vi "StartUp Sequence Open Loop Rev 1.1.vi"() -> ()   [LabVIEW 2017]
panel:
  in  "Shut Off":bool
  out "ECU COM Port Out":refnum<visa-resource-name>
  out "Throttle Position":string
  out "Turbine RPM":string
  out "Turbine Temp":string
  out "Pump Voltage":string
  out "Error Out":errorcluster
  in  "Error In":errorcluster
  in  "ECU COM Port":refnum<visa-resource-name>
  out "Turbine State":string
  in  "Strt Sqnc":bool
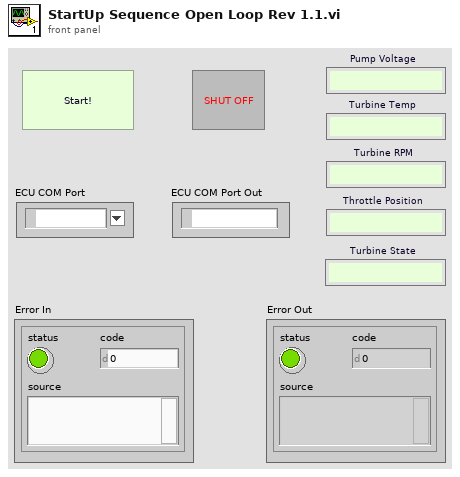
[diagram p1: front panel]
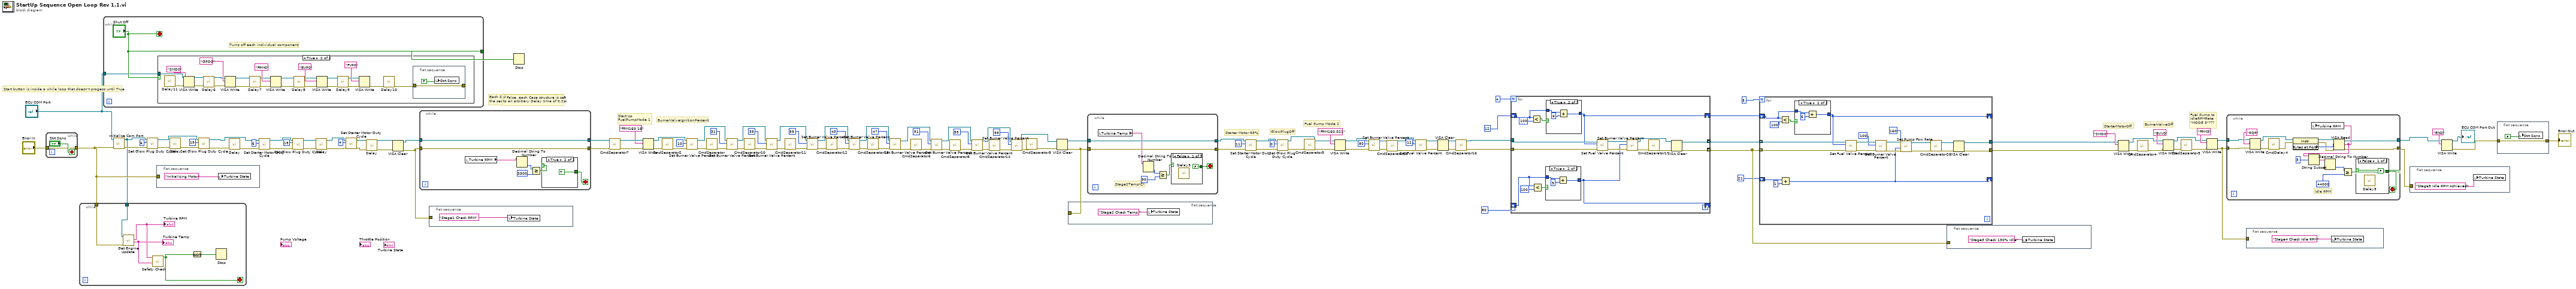
[diagram p0: block diagram]
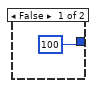
[diagram p2: hidden frame]
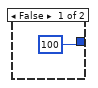
[diagram p3: hidden frame]
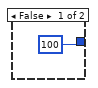
[diagram p4: hidden frame]
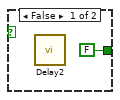
[diagram p6: hidden frame]
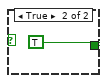
[diagram p7: hidden frame]
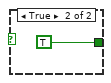
[diagram p8: hidden frame]
diagram:
  # "Start button is inside a while loop that doesn't progess until True"
  # "Fuel Pump Mode 2"
  # "Starter Motor 55%"
  # "Fuel Pump to \nIdleRPMRate\n\"MODE 3\"???"
  # "BurnerValveOff"
  # "StarterMotorOff"
  # "GlowPlugOff"
  # "Start Up\nFuelPumpMode 1"
  # "BurnerValveIgnitionPercent"
  # "If False, each Case structure is set\nto an arbitrary Delay time of 0.2 s"
  # "Each Stage is inside a while loop so that \nthe sequence doesn't progress until True"
  n1 = while {
    tunnel: "Error In" -> [w122]
    tunnel: [w122] -> w2
    stop <- "Strt Sqnc" stop-if-true
  }
  n2 = while {
    tunnel: ["Shut Off"] -> w94
    tunnel: "ECU COM Port" -> [w124]
    stop <- "Shut Off" stop-if-true
    # "Turns off each individual component"
    n3 = case shown="True" "Shut Off" {
      tunnel: w124 -> [_ w128]
      frame False {
      }
      frame True {
        n4 = call "Delay11"() -> ("error out"=w126:errorcluster)  [unwired: 11 in]
        n5 = VISA Write(VISA resource name=w128, write buffer="SMD0", error in (no error)=w126) -> (VISA resource name out=w133:refnum<visa-resource-name>, error out=w146:errorcluster)  [unwired: 1 out]
        n6 = call "Delay6"("error in (no error)"=w146) -> ("error out"=w140:errorcluster)  [unwired: 10 in]
        n7 = VISA Write(VISA resource name=w133, write buffer="GPD0", error in (no error)=w140) -> (VISA resource name out=w131:refnum<visa-resource-name>, error out=w144:errorcluster)  [unwired: 1 out]
        n8 = call "Delay7"("error in (no error)"=w144) -> ("error out"=w139:errorcluster)  [unwired: 10 in]
        n9 = VISA Write(VISA resource name=w131, write buffer="FPM0", error in (no error)=w139) -> (VISA resource name out=w130:refnum<visa-resource-name>, error out=w143:errorcluster)  [unwired: 1 out]
        n10 = call "Delay8"("error in (no error)"=w143) -> ("error out"=w138:errorcluster)  [unwired: 10 in]
        n11 = VISA Write(VISA resource name=w130, write buffer="BVP0", error in (no error)=w138) -> (VISA resource name out=w129:refnum<visa-resource-name>, error out=w142:errorcluster)  [unwired: 1 out]
        n12 = call "Delay9"("error in (no error)"=w142) -> ("error out"=w137:errorcluster)  [unwired: 10 in]
        n13 = VISA Write(VISA resource name=w129, write buffer="FVP0", error in (no error)=w137) -> (error out=w141:errorcluster)  [unwired: 2 out]
        n14 = call "Delay10"("error in (no error)"=w141) -> ("error out"=w127:errorcluster)  [unwired: 10 in]
        n15 = flat-sequence {
          tunnel: w127 -> [w147]
          tunnel: [w147] -> _
          frame #0 {
            n16 = local write "Strt Sqnc"(FALSE ("Strt Sqnc")) -> ()
          }
        }
      }
    }
  }
  n17 = call "Initialize Com Port.vi"("Error In"=w2, "ECU COM Port"="ECU COM Port") -> ("Error Out"=w82:errorcluster, "ECU COM Port Out"=w1:refnum<visa-resource-name>)  [unwired: 8 in]
  n18 = while {
    tunnel: w2 -> [w154]
    tunnel: w1 -> [w153]
    stop <- w150 stop-if-true
    n19 = call "Get Engine Update.vi"("Error In"=w154, "ECU COM Port"=w153) -> ("Temperature"=w151:string, "RPMs"=w152:string)  [unwired: 6 in, 2 out]
    "Turbine RPM" <- w152
    "Turbine Temp" <- w151
    n20 = call "Safety Check.vi"("Temperature"=w151, "RPMs"=w152) -> ("Safe?"=w150:bool)  [unwired: 9 in]
    n21 = Not(x=w150) -> (.not. x?=w149:bool)
    n22 = Stop(stop? (T)=w149) -> ()
  }
  n23 = call "Set Glow Plug Duty Cycle.vi"("Error In"=w82, "Duty Cycle"=6, "ECU COM Port"=w1) -> ("Error Out"=w81:errorcluster, "ECU COM Port Out"=w78:refnum<visa-resource-name>)  [unwired: 7 in]
  n24 = flat-sequence {
    tunnel: w2 -> [_]
    frame #0 {
      n25 = local write "Turbine State"("Initializing Motor") -> ()
    }
  }
  n26 = call "Delay"("error in (no error)"=w81) -> ("error out"=w80:errorcluster)  [unwired: 10 in]
  n27 = call "Set Glow Plug Duty Cycle.vi"("Error In"=w80, "Duty Cycle"=19, "ECU COM Port"=w78) -> ("Error Out"=w79:errorcluster, "ECU COM Port Out"=w74:refnum<visa-resource-name>)  [unwired: 7 in]
  n28 = call "Delay"("error in (no error)"=w79) -> ("error out"=w75:errorcluster)  [unwired: 10 in]
  n29 = call "Set Starter Motor Duty Cycle.vi"("Error In"=w75, "Duty Cycle"=6, "ECU COM Port"=w74) -> ("Error Out"=w73:errorcluster, "ECU COM Port Out"=w71:refnum<visa-resource-name>)  [unwired: 7 in]
  n30 = call "Set Glow Plug Duty Cycle.vi"("Error In"=w73, "Duty Cycle"=15, "ECU COM Port"=w71) -> ("Error Out"=w72:errorcluster, "ECU COM Port Out"=w67:refnum<visa-resource-name>)  [unwired: 7 in]
  n31 = call "Delay"("error in (no error)"=w72) -> ("error out"=w69:errorcluster)  [unwired: 10 in]
  n32 = call "Set Starter Motor Duty Cycle.vi"("Error In"=w69, "Duty Cycle"=4, "ECU COM Port"=w67) -> ("Error Out"=w68:errorcluster, "ECU COM Port Out"=w66:refnum<visa-resource-name>)  [unwired: 7 in]
  n33 = call "Delay"("error in (no error)"=w68) -> ("error out"=w97:errorcluster)  [unwired: 10 in]
  n34 = VISA Clear(VISA resource name=w66, error in (no error)=w97) -> (VISA resource name out=w98:refnum<visa-resource-name>, error out=w99:errorcluster)
  n35 = while {
    tunnel: w99 -> [w158]
    tunnel: w98 -> [w157]
    tunnel: [w157] -> w109
    tunnel: [w158] -> w108
    stop <- w161 stop-if-true
    n36 = local read "Turbine RPM"() -> (w156:string)
    n37 = Decimal String To Number(string=w156) -> (number=w160:i32)  [unwired: 2 in, 1 out]
    n38 = Greater Or Equal?(x=w160, y=3300) -> (x >= y?=w162:bool)
    n39 = case shown="True" w162 {
      tunnel: [FALSE TRUE] -> w161
      frame False {
        n40 = call "Delay2"() -> ()  [unwired: 11 in, 1 out]
      }
      frame True {
      }
    }
  }
  n41 = flat-sequence {
    tunnel: w99 -> [_]
    frame #0 {
      n42 = local write "Turbine State"("Stage1 Check RPM") -> ()
    }
  }
  n43 = Stop(stop? (T)=w94) -> ()
  n44 = call "CmdSeparator7"("error in (no error)"=w108) -> ("error out"=w107:errorcluster)  [unwired: 10 in]
  n45 = VISA Write(VISA resource name=w109, write buffer="FPM160,16", error in (no error)=w107) -> (VISA resource name out=w54:refnum<visa-resource-name>, error out=w120:errorcluster)  [unwired: 1 out]
  n46 = call "CmdSeparator2"("error in (no error)"=w120) -> ("error out"=w65:errorcluster)  [unwired: 10 in]
  n47 = call "Set Burner Valve Percent.vi"("Error In"=w65, "Percent"=10, "ECU COM Port"=w54) -> ("Error Out"=w64:errorcluster, "ECU COM Port Out"=w53:refnum<visa-resource-name>)  [unwired: 7 in]
  n48 = call "CmdSeparator"("error in (no error)"=w64) -> ("error out"=w63:errorcluster)  [unwired: 10 in]
  n49 = call "Set Burner Valve Percent.vi"("Error In"=w63, "Percent"=31, "ECU COM Port"=w53) -> ("Error Out"=w62:errorcluster, "ECU COM Port Out"=w52:refnum<visa-resource-name>)  [unwired: 7 in]
  n50 = call "CmdSeparator10"("error in (no error)"=w62) -> ("error out"=w61:errorcluster)  [unwired: 10 in]
  n51 = call "Set Burner Valve Percent.vi"("Error In"=w61, "Percent"=35, "ECU COM Port"=w52) -> ("Error Out"=w60:errorcluster, "ECU COM Port Out"=w51:refnum<visa-resource-name>)  [unwired: 7 in]
  n52 = call "CmdSeparator11"("error in (no error)"=w60) -> ("error out"=w59:errorcluster)  [unwired: 10 in]
  n53 = call "Set Burner Valve Percent.vi"("Error In"=w59, "Percent"=39, "ECU COM Port"=w51) -> ("Error Out"=w58:errorcluster, "ECU COM Port Out"=w50:refnum<visa-resource-name>)  [unwired: 7 in]
  n54 = call "CmdSeparator12"("error in (no error)"=w58) -> ("error out"=w57:errorcluster)  [unwired: 10 in]
  n55 = call "Set Burner Valve Percent.vi"("Error In"=w57, "Percent"=43, "ECU COM Port"=w50) -> ("Error Out"=w56:errorcluster, "ECU COM Port Out"=w49:refnum<visa-resource-name>)  [unwired: 7 in]
  n56 = call "CmdSeparator13"("error in (no error)"=w56) -> ("error out"=w55:errorcluster)  [unwired: 10 in]
  n57 = call "Set Burner Valve Percent.vi"("Error In"=w55, "Percent"=47, "ECU COM Port"=w49) -> ("Error Out"=w25:errorcluster, "ECU COM Port Out"=w24:refnum<visa-resource-name>)  [unwired: 7 in]
  n58 = call "CmdSeparator6"("error in (no error)"=w25) -> ("error out"=w27:errorcluster)  [unwired: 10 in]
  n59 = call "Set Burner Valve Percent.vi"("Error In"=w27, "Percent"=51, "ECU COM Port"=w24) -> ("Error Out"=w20:errorcluster, "ECU COM Port Out"=w21:refnum<visa-resource-name>)  [unwired: 7 in]
  n60 = call "CmdSeparator8"("error in (no error)"=w20) -> ("error out"=w23:errorcluster)  [unwired: 10 in]
  n61 = call "Set Burner Valve Percent.vi"("Error In"=w23, "Percent"=55, "ECU COM Port"=w21) -> ("Error Out"=w16:errorcluster, "ECU COM Port Out"=w17:refnum<visa-resource-name>)  [unwired: 7 in]
  n62 = call "CmdSeparator14"("error in (no error)"=w16) -> ("error out"=w19:errorcluster)  [unwired: 10 in]
  n63 = call "Set Burner Valve Percent.vi"("Error In"=w19, "Percent"=59, "ECU COM Port"=w17) -> ("Error Out"=w15:errorcluster, "ECU COM Port Out"=w14:refnum<visa-resource-name>)  [unwired: 7 in]
  n64 = call "CmdSeparator9"("error in (no error)"=w15) -> ("error out"=w93:errorcluster)  [unwired: 10 in]
  n65 = VISA Clear(VISA resource name=w14, error in (no error)=w93) -> (VISA resource name out=w95:refnum<visa-resource-name>, error out=w96:errorcluster)
  n66 = flat-sequence {
    tunnel: w96 -> [_]
    frame #0 {
      n67 = local write "Turbine State"("Stage2 Check Temp.") -> ()
    }
  }
  n68 = while {
    tunnel: w95 -> [w168]
    tunnel: w96 -> [w169]
    tunnel: [w168] -> w36
    tunnel: [w169] -> w38
    stop <- w172 stop-if-true
    # "Stage2Temp(C)"
    n69 = local read "Turbine Temp"() -> (w167:string)
    n70 = Decimal String To Number(string=w167) -> (number=w170:i32)  [unwired: 2 in, 1 out]
    n71 = Greater Or Equal?(x=w170, y=90) -> (x >= y?=w173:bool)
    n72 = case shown="False" w173 {
      tunnel: [FALSE TRUE] -> w172
      frame False {
        n73 = call "Delay3"() -> ()  [unwired: 11 in, 1 out]
      }
      frame True {
      }
    }
  }
  n74 = call "Set Starter Motor Duty Cycle.vi"("Error In"=w38, "Duty Cycle"=11, "ECU COM Port"=w36) -> ("Error Out"=w37:errorcluster, "ECU COM Port Out"=w35:refnum<visa-resource-name>)  [unwired: 7 in]
  n75 = call "Set Glow Plug Duty Cycle.vi"("Error In"=w37, "Duty Cycle"=0, "ECU COM Port"=w35) -> ("Error Out"=w34:errorcluster, "ECU COM Port Out"=w32:refnum<visa-resource-name>)  [unwired: 7 in]
  n76 = call "CmdSeparator3"("error in (no error)"=w34) -> ("error out"=w33:errorcluster)  [unwired: 10 in]
  n77 = VISA Write(VISA resource name=w32, write buffer="FPM160,021", error in (no error)=w33) -> (VISA resource name out=w29:refnum<visa-resource-name>, error out=w31:errorcluster)  [unwired: 1 out]
  n78 = call "Set Burner Valve Percent.vi"("Error In"=w31, "Percent"=80, "ECU COM Port"=w29) -> ("Error Out"=w13:errorcluster, "ECU COM Port Out"=w28:refnum<visa-resource-name>)  [unwired: 7 in]
  n79 = call "CmdSeparator18"("error in (no error)"=w13) -> ("error out"=w12:errorcluster)  [unwired: 10 in]
  n80 = call "Set Fuel Valve Percent.vi"("Error In"=w12, "Percent"=12, "ECU COM Port"=w28) -> ("Error Out"=w11:errorcluster, "ECU COM Port Out"=w30:refnum<visa-resource-name>)  [unwired: 7 in]
  n81 = VISA Clear(VISA resource name=w30, error in (no error)=w11) -> (VISA resource name out=w89:refnum<visa-resource-name>, error out=w90:errorcluster)
  n82 = call "CmdSeparator16"("error in (no error)"=w90) -> ("error out"=w88:errorcluster)  [unwired: 10 in]
  n83 = for {
    N: 4 -> [_]
    tunnel: [w176] -> _
    tunnel: [w177] -> _
    tunnel: w89 -> [w184]
    tunnel: w88 -> [w185]
    shift-right: [w183] -> w6
    shift-left: 12 -> [w189]
    shift-right: [w180] -> _
    shift-left: 80 -> [w186]
    tunnel: [w177] -> w8 mode=indexing
    tunnel: [w176] -> w7 mode=indexing
    n84 = Less?(x=w189, y=100) -> (x < y?=w190:bool)
    n85 = Less?(x=w186, y=100) -> (x < y?=w187:bool)
    n86 = case shown="True" w187 {
      tunnel: w186 -> [_ w196]
      tunnel: [100 w194] -> w180
      frame False {
      }
      frame True {
        n87 = Add(x=w196, y=5) -> (x+y=w194:i32)
      }
    }
    n88 = case shown="True" w190 {
      tunnel: w189 -> [_ w200]
      tunnel: [100 w198] -> w183
      frame False {
      }
      frame True {
        n89 = Add(x=w200, y=6) -> (x+y=w198:i32)
      }
    }
    n90 = call "Set Fuel Valve Percent.vi"("Error In"=w185, "Percent"=w183, "ECU COM Port"=w184) -> ("Error Out"=w182:errorcluster, "ECU COM Port Out"=w179:refnum<visa-resource-name>)  [unwired: 7 in]
    n91 = call "Set Burner Valve Percent.vi"("Error In"=w182, "Percent"=w180, "ECU COM Port"=w179) -> ("Error Out"=w181:errorcluster, "ECU COM Port Out"=w178:refnum<visa-resource-name>)  [unwired: 7 in]
    n92 = call "CmdSeparator17"("error in (no error)"=w181) -> ("error out"=w192:errorcluster)  [unwired: 10 in]
    n93 = VISA Clear(VISA resource name=w178, error in (no error)=w192) -> (VISA resource name out=w176:refnum<visa-resource-name>, error out=w177:errorcluster)
  }
  n94 = for {
    N: 5 -> [_]
    tunnel: [w212] -> w3
    tunnel: [w213] -> w4
    shift-right: [w216] -> _
    shift-left: w6 -> [w217]
    tunnel: w8 -> [w211] mode=indexing
    tunnel: w7 -> [w210] mode=indexing
    shift-right: [w201] -> _
    shift-left: 21 -> [w202]
    n95 = Less?(x=w217, y=100) -> (x < y?=w218:bool)
    n96 = Add(x=w202, y=1) -> (x+y=w201:i32)
    n97 = case shown="True" w218 {
      tunnel: w217 -> [_ w224]
      tunnel: [100 w222] -> w216
      frame False {
      }
      frame True {
        n98 = Add(x=w224, y=6) -> (x+y=w222:i32)
      }
    }
    n99 = call "Set Fuel Valve Percent.vi"("Error In"=w211, "Percent"=w216, "ECU COM Port"=w210) -> ("Error Out"=w215:errorcluster, "ECU COM Port Out"=w214:refnum<visa-resource-name>)  [unwired: 7 in]
    n100 = call "Set Burner Valve Percent.vi"("Error In"=w215, "Percent"=100 ("y"), "ECU COM Port"=w214) -> ("Error Out"=w205:errorcluster, "ECU COM Port Out"=w208:refnum<visa-resource-name>)  [unwired: 7 in]
    n101 = call "Set Pump Fow Rate.vi"("Error In"=w205, "Pulse Width"=w201, "Voltage"=160 ("y"), "ECU COM Port"=w208) -> ("Error Out"=w206:errorcluster, "ECU COM Port Out"=w207:refnum<visa-resource-name>)  [unwired: 6 in]
    n102 = call "CmdSeparator20"("error in (no error)"=w206) -> ("error out"=w220:errorcluster)  [unwired: 10 in]
    n103 = VISA Clear(VISA resource name=w207, error in (no error)=w220) -> (VISA resource name out=w212:refnum<visa-resource-name>, error out=w213:errorcluster)
  }
  n104 = flat-sequence {
    tunnel: w8 -> [_]
    frame #0 {
      n105 = local write "Turbine State"("Stage3 Check 130% Idle") -> ()
    }
  }
  n106 = VISA Write(VISA resource name=w3, write buffer="SMD0", error in (no error)=w4) -> (VISA resource name out=w115:refnum<visa-resource-name>, error out=w117:errorcluster)  [unwired: 1 out]
  n107 = call "CmdSeparator4"("error in (no error)"=w117) -> ("error out"=w116:errorcluster)  [unwired: 10 in]
  n108 = VISA Write(VISA resource name=w115, write buffer="BVV0", error in (no error)=w116) -> (VISA resource name out=w112:refnum<visa-resource-name>, error out=w111:errorcluster)  [unwired: 1 out]
  n109 = call "CmdSeparator5"("error in (no error)"=w111) -> ("error out"=w113:errorcluster)  [unwired: 10 in]
  n110 = VISA Write(VISA resource name=w112, write buffer="FPM3", error in (no error)=w113) -> (VISA resource name out=w110:refnum<visa-resource-name>, error out=w101:errorcluster)  [unwired: 1 out]
  n111 = while {
    tunnel: w110 -> [w232]
    tunnel: w101 -> [w231]
    tunnel: [w229] -> w100
    tunnel: [w228] -> w103
    stop <- w243 stop-if-true
    # "Idle RPM"
    n112 = VISA Write(VISA resource name=w232, write buffer="RQR", error in (no error)=w231) -> (VISA resource name out=w239:refnum<visa-resource-name>, error out=w241:errorcluster)  [unwired: 1 out]
    n113 = call "CmdDelay4"("error in (no error)"=w241) -> ("error out"=w240:errorcluster)  [unwired: 10 in]
    n114 = property class="Instr"(reference=w239, error in=w240) -> (reference out=w236:refnum<visa-resource-name>, error out=w237:errorcluster, "Bytes at Port"=w238:u32)
    n115 = VISA Read(VISA resource name=w236, byte count=w238, error in (no error)=w237) -> (VISA resource name out=w228:refnum<visa-resource-name>, read buffer=w230:string, error out=w229:errorcluster)  [unwired: 1 out]
    n116 = String Subset(string=w230, offset (0)=3) -> (substring=w234:string)  [unwired: 1 in]
    n117 = local write "Turbine RPM"(w230) -> ()
    n118 = Decimal String To Number(string=w234) -> (number=w233:i32)  [unwired: 2 in, 1 out]
    n119 = Greater Or Equal?(x=w233, y=44000) -> (x >= y?=w227:bool)
    n120 = case shown="False" w227 {
      tunnel: [FALSE TRUE] -> w243
      frame False {
        n121 = call "Delay5"() -> ()  [unwired: 11 in, 1 out]
      }
      frame True {
      }
    }
  }
  n122 = flat-sequence {
    tunnel: w101 -> [_]
    frame #0 {
      n123 = local write "Turbine State"("Stage4 Check Idle RPM") -> ()
    }
  }
  n124 = flat-sequence {
    tunnel: w100 -> [_]
    frame #0 {
      n125 = local write "Turbine State"("Stage5 Idle RPM Achieved") -> ()
    }
  }
  n126 = VISA Write(VISA resource name=w103, write buffer="END") -> (VISA resource name out=→"ECU COM Port Out":refnum<visa-resource-name>, error out=w92:errorcluster)  [unwired: 1 in, 1 out]
  n127 = flat-sequence {
    tunnel: w92 -> [w248]
    tunnel: [w248] -> w91
    frame #0 {
      n128 = local write "Strt Sqnc"(FALSE ("Strt Sqnc")) -> ()
    }
  }
  "Error Out" <- w91
